vi "AsyncResp-Background-Thread.vi"(7 "TcpRouter-Client":refnum<class "TcpRouter-Client.lvclass">, 8 "error in (no error)":errorcluster) -> (0 "error out":errorcluster)   [LabVIEW 2020, in "CSM-TCP-Router.lvlib" / "TcpRouter-Client.lvclass"]
uses:
  TcpRouter-Client.lvclass
  TcpRouter-Client.lvclass/TcpRouter-Client.ctl
  Def-TCP-Router Async-Resp Data.ctl
  CSM-TCP-Router.lvlib
  <userlib>/_NEVSTOP/Communicable State Machine(CSM)/_Shared/CSM Shared.lvlib
panel:
  out "current time":timestamp
  out "String":string
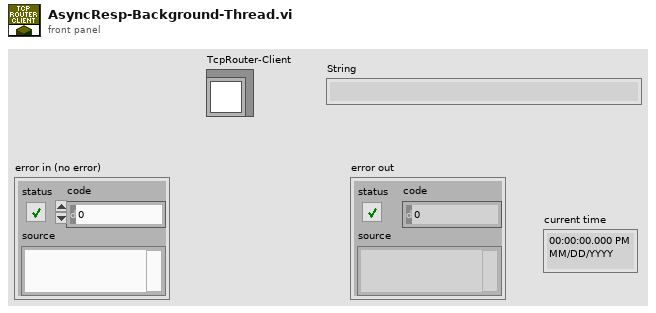
[diagram p1: front panel]
types:
  T1 = typedef "CSM-TCP-Router.lvlib/TcpRouter-Client.lvclass/Def-TCP-Router Async-Resp Data.ctl" = cluster{"status":string, "arg":string, "source":string, "error":errorcluster}
  T2 = typedef "CSM-TCP-Router.lvlib/TcpRouter-Client.lvclass/Def-TCP-Router ASYNC-RESP.ctl" = cluster{"Async-Resp":refnum<k5>, "RespQueue":refnum<queue>, "RespEvent":refnum<user-event>}
  T3 = typedef "CSM-TCP-Router.lvlib/tcp-msg type.ctl" = enum8{"info", "error", "cmd", "cmd-resp", "resp", "async-resp", "status", "interrupt"}
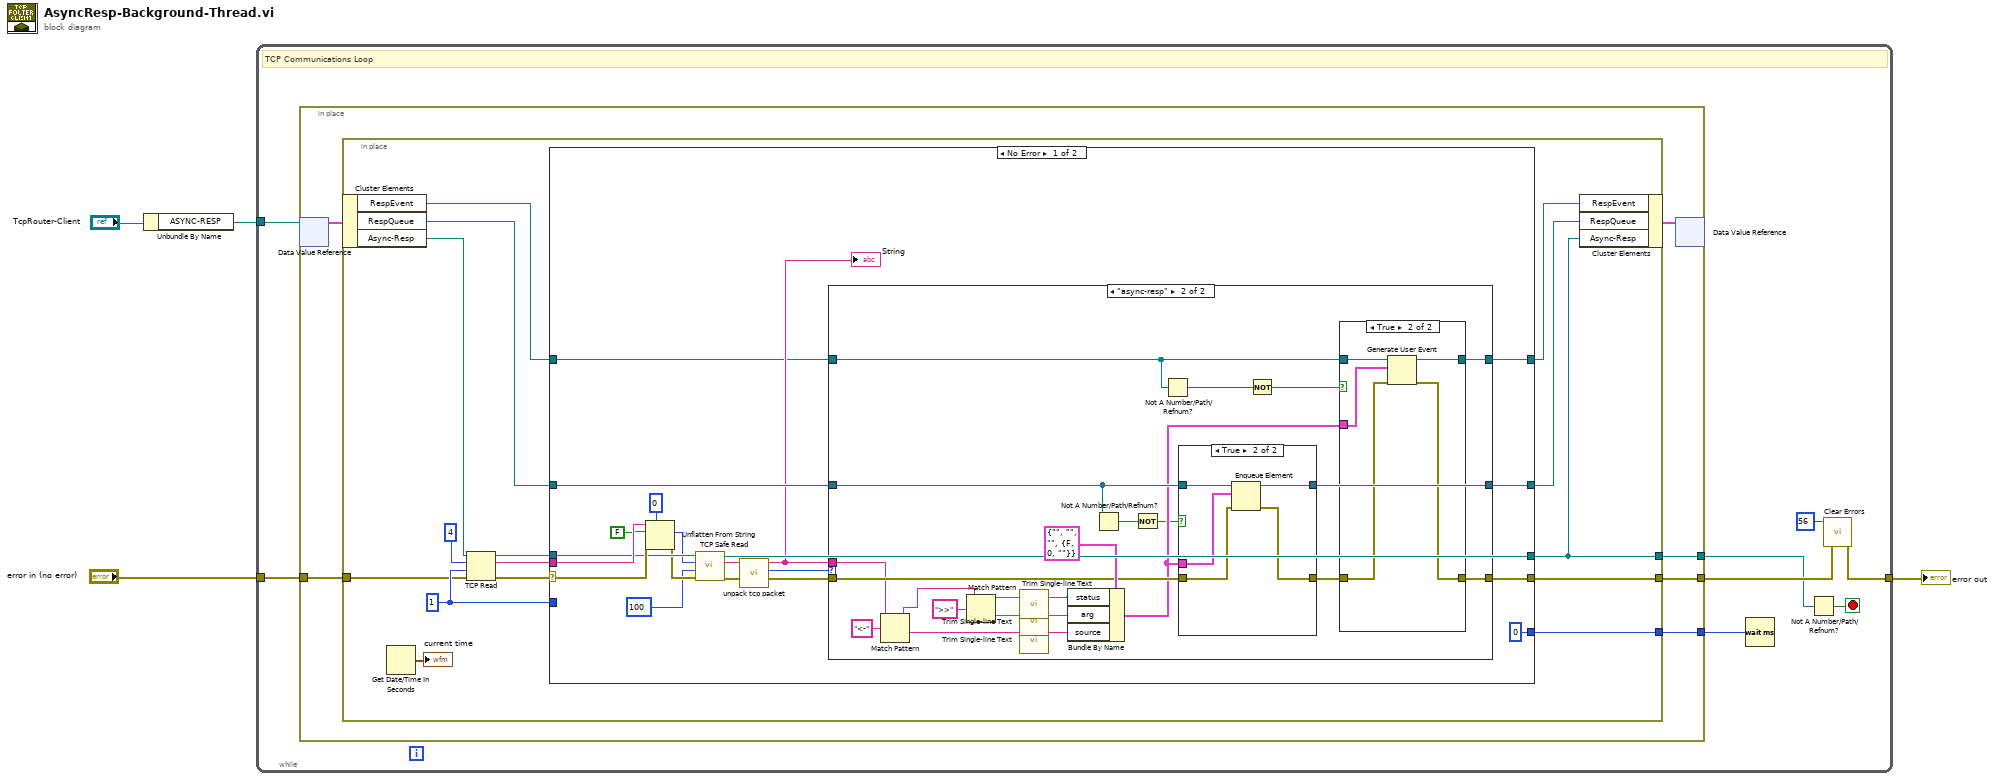
[diagram p0: block diagram]
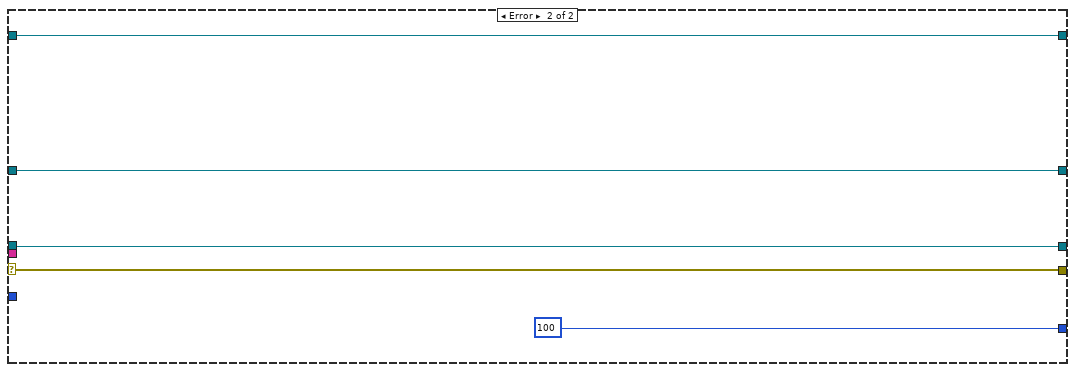
[diagram p5: hidden frame]
diagram:
  n1 = Unbundle By Name("TcpRouter-Client") -> ("ASYNC-RESP"=w1:refnum<data-value>)
  n2 = while {
    tunnel: [w11] -> w3
    tunnel: "error in (no error)" -> [w8]
    tunnel: w1 -> [w9]
    stop <- w10 stop-if-true
    # "TCP Communications Loop"
    n3 = in-place {
      in-place-border: w8 -> [w16]
      in-place-border: [w15] -> w7
      in-place-border: [w14] -> w6
      in-place-border: [w13] -> w5
      n4 = in-place-dvr #1(w9) -> (w18:T2)  [unwired: 1 out]
      n5 = in-place {
        in-place-border: w16 -> [w25]
        in-place-border: [w24] -> w15
        in-place-border: [w23] -> w14
        in-place-border: [w22] -> w13
        w29 = 1 ("timeout ms (1000)")
        n6 = in-place-cluster #2(w18) -> ("RespEvent"=w20:refnum<user-event>, "RespQueue"=w28:refnum<queue>, "Async-Resp"=w26:refnum<k5>)
        n7 = Get Date/Time In Seconds() -> (seconds since 1Jan1904=→"current time":timestamp)
        n8 = TCP Read(connection ID=w26, bytes to read=4, error in (no error)=w25, 9:w29) -> (connection ID out=w31:refnum<k5>, data out=w32:string, error out=w33:errorcluster)  [unwired: 1 in]
        n9 = case shown="No Error" w33 {
          selector: w33 -> [w50 w97]
          tunnel: [w52 w96] -> w23
          tunnel: [w40 w97] -> w24
          tunnel: [w51 w95] -> w27
          tunnel: w32 -> [w49 _]
          tunnel: w31 -> [w48 w96]
          tunnel: w29 -> [_ _]
          tunnel: w28 -> [w39 w95]
          tunnel: [u32 0 ("milliseconds to wait") u32 100 ("milliseconds to wait")] -> w22
          tunnel: w20 -> [w35 w93]
          tunnel: [w34 w93] -> w19
          frame No Error {
            n10 = Unflatten From String(type=0, binary string=w49, data includes array or string size? (T)=FALSE, error in (no error)=w50) -> (value=w46:i32, error out=w45:errorcluster)  [unwired: 2 out]
            n11 = call "TCP Safe Read.vi"("error in (no error)"=w45, "timeout ms (25000)"=100 ("timeout ms (1000)"), "bytes to read"=w46, "TCP Network Connection in"=w48) -> ("error out"=w41:errorcluster, "String"=w47:string, "TCP Network Connection out"=w52:refnum<k5>)  [unwired: 5 in]
            n12 = call "unpack tcp packet.vi"("TCP Pack"=w47) -> ("tcp-message-type"=w42:T3, "String"=w36:string)  [unwired: 9 in]
            "String" <- w36
            n13 = case shown="\"async-resp\"" w42 {
              tunnel: [w54 w78] -> w51
              tunnel: w36 -> [_ w73]
              tunnel: w41 -> [w55 w76]
              tunnel: [w55 w60] -> w40
              tunnel: w39 -> [w54 w75]
              tunnel: w35 -> [w53 w63]
              tunnel: [w53 w62] -> w34
              frame Default {
              }
              frame "async-resp" {
                n14 = Match Pattern(string=w73, regular expression="<-") -> (before substring=w69:string, after substring=w71:string)  [unwired: 1 in, 2 out]
                n15 = Match Pattern(string=w69, regular expression=">>") -> (before substring=w68:string, after substring=w67:string)  [unwired: 1 in, 2 out]
                n16 = call <userlib>:"Trim Single-line Text.vi"("single-line text"=w68) -> ("trimed text"=w64:string)  [unwired: 2 in]
                n17 = call <userlib>:"Trim Single-line Text.vi"("single-line text"=w67) -> ("trimed text"=w65:string)  [unwired: 2 in]
                n18 = call <userlib>:"Trim Single-line Text.vi"("single-line text"=w71) -> ("trimed text"=w70:string)  [unwired: 2 in]
                n19 = Bundle By Name(cluster=T1 {"status"="", "arg"="", "source"="", "error"={"status"=FALSE, "code"=0, "source"=""}} ("Cluster"), "status"=w64, "arg"=w65, "source"=w70) -> (w58:T1)
                n20 = Not A Number/Path/Refnum?(number/path/refnum=w75) -> (NaN/Path/Refnum?=w74:bool)
                n21 = Not(x=w74) -> (.not. x?=w56:bool)
                n22 = Not A Number/Path/Refnum?(number/path/refnum=w63) -> (NaN/Path/Refnum?=w59:bool)
                n23 = case shown="True" w56 {
                  tunnel: [w87 w92] -> w78
                  tunnel: w58 -> [_ w91]
                  tunnel: w76 -> [w86 w90]
                  tunnel: [w86 w89] -> w61
                  tunnel: w75 -> [w87 w88]
                  frame False {
                  }
                  frame True {
                    n24 = Enqueue Element(queue=w88, element=w91, error in (no error)=w90) -> (queue out=w92:refnum<queue>, error out=w89:errorcluster)  [unwired: 1 in, 1 out]
                  }
                }
                n25 = Not(x=w59) -> (.not. x?=w57:bool)
                n26 = case shown="True" w57 {
                  tunnel: w63 -> [w80 w85]
                  tunnel: [w80 w84] -> w62
                  tunnel: w61 -> [w79 w83]
                  tunnel: [w79 w82] -> w60
                  tunnel: w58 -> [_ w81]
                  frame False {
                  }
                  frame True {
                    n27 = Generate User Event(user event=w85, event data cluster=w81, error in=w83) -> (user event out=w84:refnum<user-event>, error out=w82:errorcluster)  [unwired: 1 in]
                  }
                }
              }
            }
          }
          frame Error {
          }
        }
        n28 = in-place-cluster #2("RespEvent"=w19, "RespQueue"=w27, "Async-Resp"=w23) -> (w17:T2)
      }
      n29 = in-place-dvr #1(w17) -> ()  [unwired: 2 out]
    }
    n30 = Wait (ms)(milliseconds to wait=w5) -> ()  [unwired: 1 out]
    n31 = Not A Number/Path/Refnum?(number/path/refnum=w6) -> (NaN/Path/Refnum?=w10:bool)
    n32 = call <vilib>:"Clear Errors.vi"("error in (no error)"=w7, "specific error code to clear (0: all)"=56) -> ("error out"=w11:errorcluster)  [unwired: 4 in, 1 out]
  }
  "error out" <- w3
